vi "base64 decode.vi"(1 "base64 encoded string":string) -> (0 "decoded data":u8[](array[numeric]) format="%.0x")   [LabVIEW 2019, in "WebSocket Server Toolkit.lvlib"]
uses:
  WebSocket Server Toolkit.lvlib
  char to binary.ctl
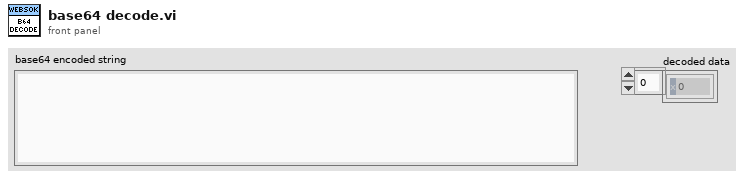
[diagram p1: front panel]
types:
  T1 = typedef "WebSocket Server Toolkit.lvlib/char to binary.ctl" = map{u8, u8}
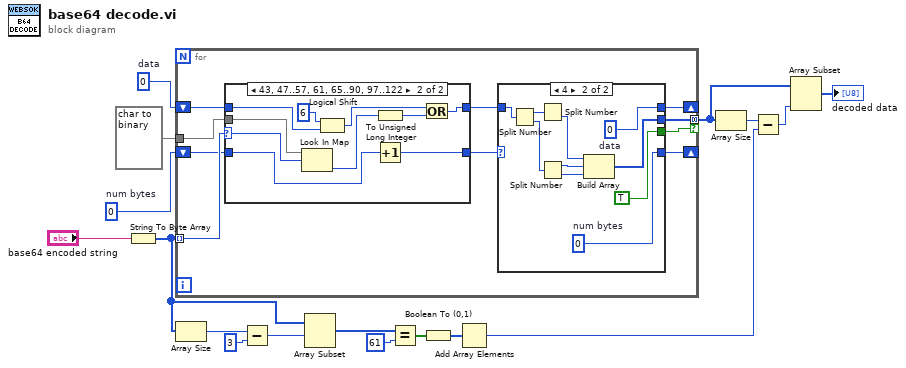
[diagram p0: block diagram]
diagram:
  w7 = u32 0  # num bytes
  w8 = u32 0  # data
  n1 = String To Byte Array(string="base64 encoded string") -> (unsigned byte array=w9:u8[])
  n2 = for {
    tunnel: w9 -> [w26] mode=indexing
    shift-right: [w18] -> _
    shift-left: w8 -> [w25]
    shift-right: [w19] -> _
    shift-left: w7 -> [w24]
    tunnel: T1 {43=62, 47=63, 48=52, 49=53, 50=54, 51=55, 52=56, 53=57, 54=58, 55=59, 56=60, 57=61, 65=0, 66=1, 67=2, 68=3, 69=4, 70=5, 71=6, 72=7, 73=8, 74=9, 75=10, 76=11, 77=12, 78=13, 79=14, 80=15, 81=16, 82=17, 83=18, 84=19, 85=20, 86=21, 87=22, 88=23, 89=24, 90=25, 97=26, 98=27, 99=28, 100=29, 101=30, 102=31, 103=32, 104=33, 105=34, 106=35, 107=36, 108=37, 109=38, 110=39, 111=40, 112=41, 113=42, 114=43, 115=44, 116=45, 117=46, 118=47, 119=48, 120=49, 121=50, 122=51} ("char to binary") -> [w27]
    tunnel: [w21] -> w3 mode=concatenating if=w20
    n3 = case shown="43, 47..57, 61, 65..90, 97..122" w26 {
      selector: w26 -> [_ w50]
      tunnel: w27 -> [_ w51]
      tunnel: w25 -> [w40 w48]
      tunnel: w24 -> [w41 w44]
      tunnel: [w41 w43] -> w23
      tunnel: [w40 w42] -> w22
      frame Default {
      }
      frame 43, 47..57, 61, 65..90, 97..122 {
        n4 = Look In Map(map=w51, key=w50) -> (value=w47:u8)  [unwired: 1 in, 1 out]
        n5 = Logical Shift(y=i16 6, x=w48) -> (x << y=w46:u32)
        n6 = To Unsigned Long Integer(number=w47) -> (unsigned 32bit integer=w45:u32)
        n7 = Increment(x=w44) -> (x+1=w43:u32)
        n8 = Or(x=w46, y=w45) -> (x .or. y?=w42:u32)
      }
    }
    n9 = case shown="4" w23 {
      selector: w23 -> [w29 _]
      tunnel: w22 -> [w28 w34]
      tunnel: [_ w33] -> w21
      tunnel: [_ TRUE] -> w20
      tunnel: [w29 w31] -> w19
      tunnel: [w28 w30] -> w18
      frame Default {
      }
      frame 4 {
        w30 = u32 0  # data
        w31 = u32 0  # num bytes
        n10 = Split Number(x=w34) -> (hi(x)=w38:u16, lo(x)=w39:u16)
        n11 = Split Number(x=w38) -> (lo(x)=w37:u8)  [unwired: 1 out]
        n12 = Split Number(x=w39) -> (hi(x)=w35:u8, lo(x)=w36:u8)
        n13 = Build Array(w37, w35, w36) -> (w33:u8[])
      }
    }
  }
  n14 = Array Size(array=w9) -> (size(s)=w16:i32)
  n15 = Subtract(x=w16, y=3) -> (x-y=w14:i32)
  n16 = Array Subset(array=w9, index=w14) -> (w13:u8[])  [unwired: 1 in]
  n17 = Equal?(x=w13, y=u8 61) -> (x = y?=w11:bool[])
  n18 = Boolean To (0,1)(Boolean=w11) -> (0, 1=w10:i16[])
  n19 = Add Array Elements(numeric array=w10) -> (sum=w2:i16)
  n20 = Array Size(array=w3) -> (size(s)=w4:i32)
  n21 = Subtract(x=w4, y=w2) -> (x-y=w5:i32)
  n22 = Array Subset(array=w3, length=w5) -> (→"decoded data":u8[])  [unwired: 1 in]
